vi "BfieldPreRunGraph_DP_Ver1.0.vi"(0 "B Array":dbl[](array[numeric]), 2 "Set Pt":dbl) -> (5 "BField Graph":dbl[][](graph))   [LabVIEW 2012]
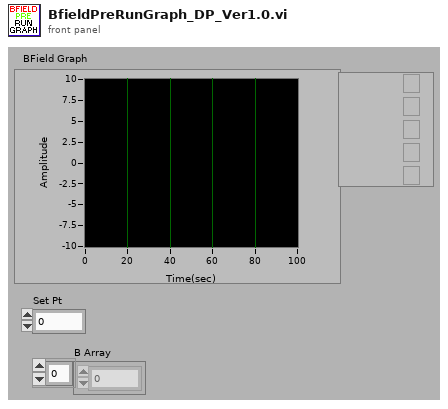
[diagram p1: front panel]
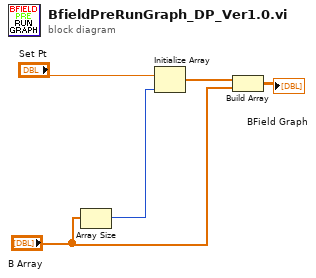
[diagram p0: block diagram]
diagram:
  n1 = Array Size(array="B Array") -> (size(s)=w5:i32)
  n2 = Initialize Array("Set Pt", w5) -> (w3:dbl[])
  n3 = Build Array(w3, "B Array") -> (→"BField Graph":dbl[][])
